vi "hello_world.vi"() -> ()   [LabVIEW 2015]
panel:
  out "String":string="hello world"
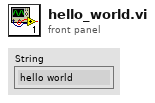
[diagram p1: front panel]
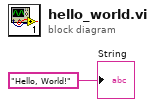
[diagram p0: block diagram]
diagram:
  "String" <- "Hello, World!"
